vi "Motor Stop.vi"(8 "error in (no error)":errorcluster, 11 "ZanClass in":refnum<class "ZanClass.lvclass">) -> (0 "error out":errorcluster, 3 "ZanClass out":refnum<class "ZanClass.lvclass">)   [LabVIEW 2019, in "ZanClass.lvclass"]
uses:
  ZanClass.lvclass
  LLB/zmotion/zaux/zauxdll.lvlib
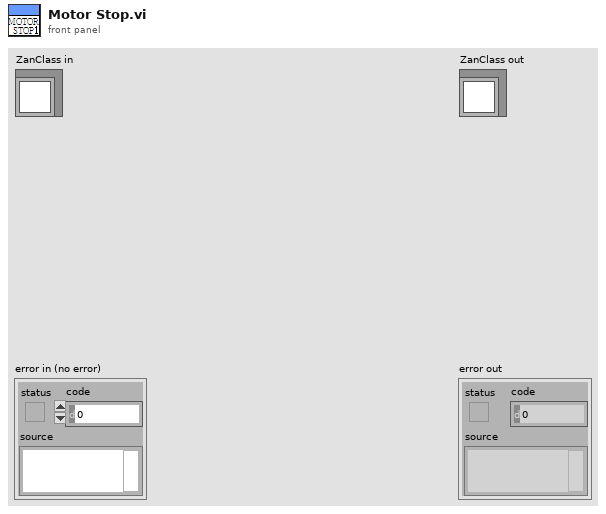
[diagram p1: front panel]
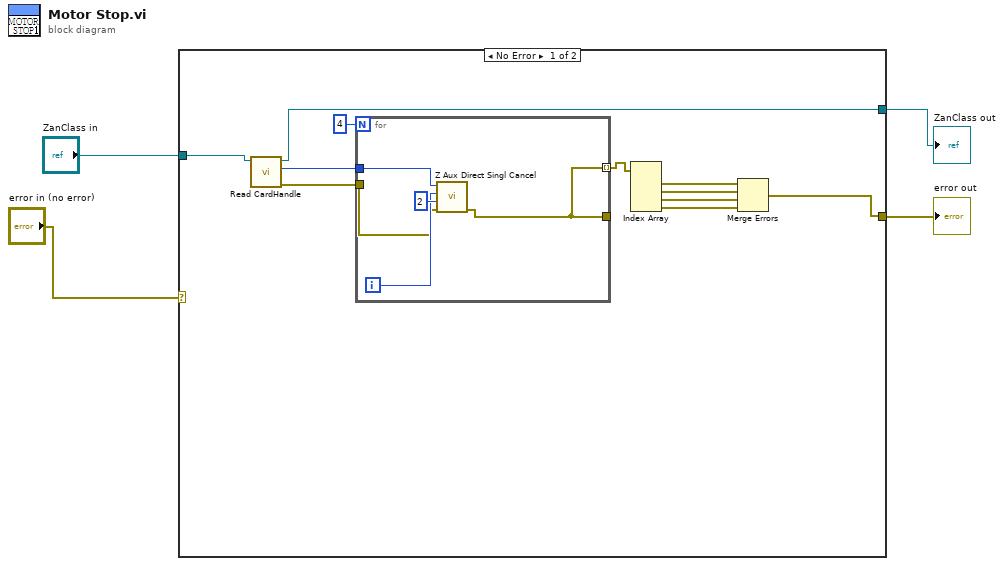
[diagram p0: block diagram]
diagram:
  n1 = case shown="No Error" "error in (no error)" {
    selector: "error in (no error)" -> [_ w21]
    tunnel: "ZanClass in" -> [w15 w22]
    tunnel: [w12 w22] -> w2
    tunnel: [w5 w21] -> w1
    frame No Error {
      n2 = call-dynamic "Read CardHandle.vi"("AxisCard in"=w15) -> ("error out"=w11:errorcluster, "CardHandle"=w14:i32, "AxisCard out"=w12:refnum<class "ZanClass.lvclass">)  [unwired: 8 in]
      n3 = for {
        N: 4 -> [_]
        tunnel: w14 -> [w20]
        tunnel: w11 -> [w17]
        tunnel: [w16] -> _
        tunnel: [w16] -> w10 mode=indexing
        i -> [w18]
        n4 = call "Z Aux Direct Singl Cancel.vi"("error in (no error)"=w17, "imode"=2, "iaxis"=w18, "handle"=w20) -> ("error out"=w16:errorcluster)  [unwired: 5 in, 2 out]
      }
      n5 = Index Array(array=w10) -> (element #1=w9:errorcluster, element #2=w8:errorcluster, element #3=w7:errorcluster, element #4=w6:errorcluster)  [unwired: 4 in]
      n6 = Merge Errors(w9, w8, w7, w6) -> (w5:errorcluster)
    }
    frame Error {
    }
  }
  "error out" <- w1
  "ZanClass out" <- w2
